vi "IP地址二进制文件生成器.vi"() -> ()   [LabVIEW 2017]
panel:
  in  "String":string="括\n\u0014"
  in  "file (use dialog)":path
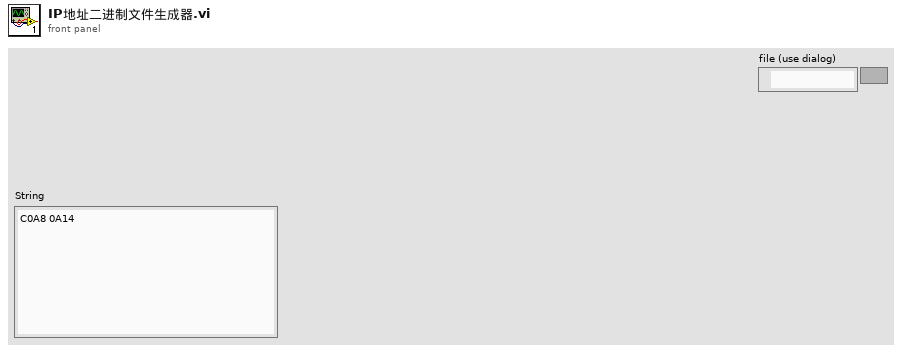
[diagram p1: front panel]
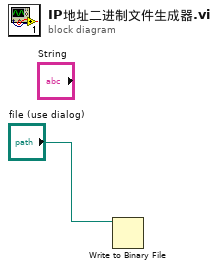
[diagram p0: block diagram]
diagram:
  n1 = Write to Binary File(file (use dialog)="file (use dialog)") -> ()  [unwired: 5 in, 3 out]
